vi "Array_filter_elements_string.vi"(10 "set2":string[](array[string]), 11 "set1":string[](array[string])) -> (1 "shared":string[](array[string]), 2 "deleted":string[](array[string]), 3 "filtered":string[](array[string]))   [LabVIEW 2019]
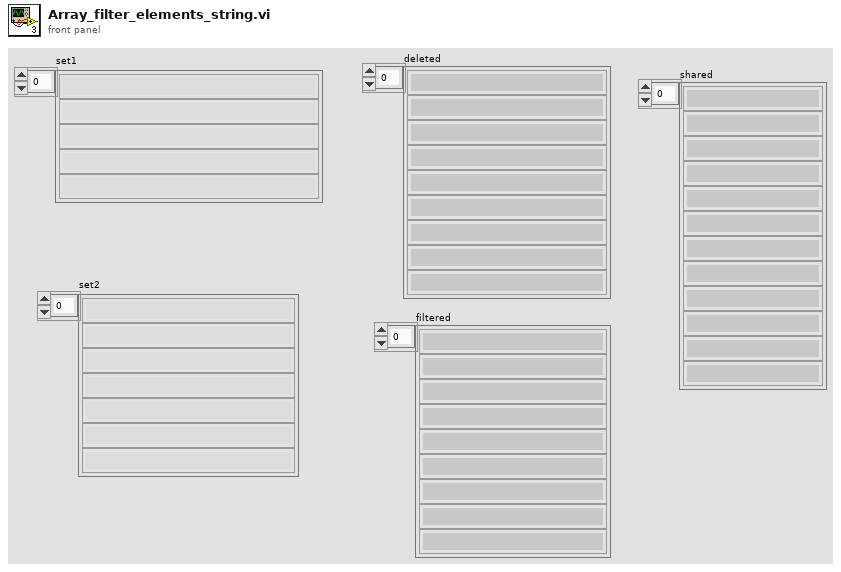
[diagram p1: front panel]
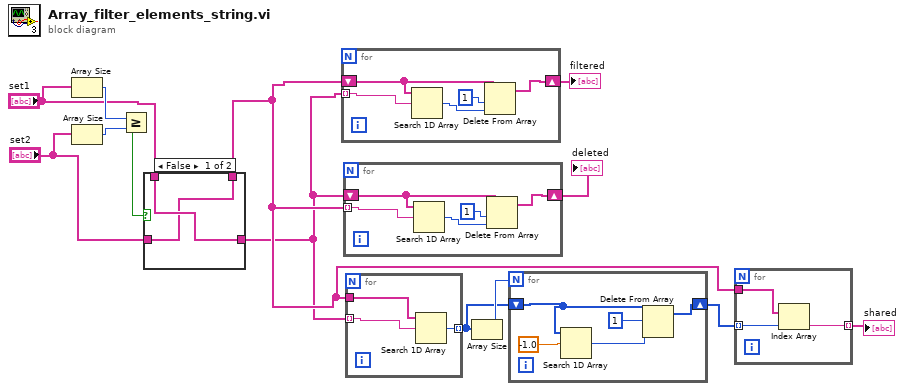
[diagram p0: block diagram]
diagram:
  n1 = Array Size(array="set1") -> (size(s)=w7:i32)
  n2 = Array Size(array="set2") -> (size(s)=w6:i32)
  n3 = Greater Or Equal?(x=w7, y=w6) -> (x >= y?=w5:bool)
  n4 = case shown="False" w5 {
    tunnel: [w14 w17] -> w3
    tunnel: "set1" -> [w15 w17]
    tunnel: "set2" -> [w14 w16]
    tunnel: [w15 w16] -> w1
    frame False {
    }
    frame True {
    }
  }
  n5 = for {
    tunnel: w1 -> [w22] mode=indexing
    shift-right: [w18] -> w13
    shift-left: w3 -> [w21]
    n6 = Search 1D Array(1D array=w21, element=w22) -> (index of element=w20:i32)  [unwired: 1 in]
    n7 = Delete From Array(array=w21, length=1, index=w20) -> (array with subset deleted=w18:string[])  [unwired: 1 out]
  }
  "filtered" <- w13
  n8 = for {
    tunnel: w3 -> [w27] mode=indexing
    shift-right: [w23] -> w12
    shift-left: w1 -> [w26]
    n9 = Search 1D Array(1D array=w26, element=w27) -> (index of element=w25:i32)  [unwired: 1 in]
    n10 = Delete From Array(array=w26, length=1, index=w25) -> (array with subset deleted=w23:string[])  [unwired: 1 out]
  }
  "deleted" <- w12
  n11 = for {
    tunnel: w1 -> [w30] mode=indexing
    tunnel: w3 -> [w29]
    tunnel: [w28] -> w8 mode=indexing
    n12 = Search 1D Array(1D array=w29, element=w30) -> (index of element=w28:i32)  [unwired: 1 in]
  }
  n13 = Array Size(array=w8) -> (size(s)=w9:i32)
  n14 = for {
    N: w9 -> [_]
    shift-right: [w31] -> w11
    shift-left: w8 -> [w32]
    n15 = Search 1D Array(1D array=w32, element=-1.0) -> (index of element=w35:i32)  [unwired: 1 in]
    n16 = Delete From Array(array=w32, length=1, index=w35) -> (array with subset deleted=w31:i32[])  [unwired: 1 out]
  }
  n17 = for {
    tunnel: w11 -> [w38] mode=indexing
    tunnel: w3 -> [w37]
    tunnel: [w36] -> w10 mode=indexing
    n18 = Index Array(array=w37, index=w38) -> (element=w36:string)
  }
  "shared" <- w10
